vi "genMotionSensorPacket.vi"(10 "node ID":u8, 11 "state":bool) -> (3 "packet string":string)   [LabVIEW 2011]
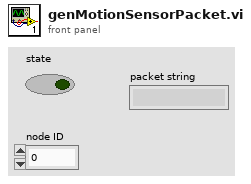
[diagram p1: front panel]
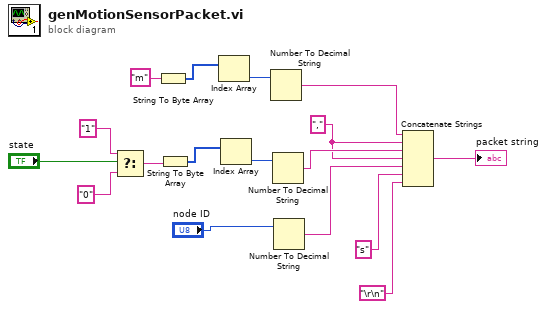
[diagram p0: block diagram]
diagram:
  w5 = ","
  n1 = Select(t="1", s="state", f="0") -> (s? t:f=w9:string)
  n2 = String To Byte Array(string="m") -> (unsigned byte array=w16:u8[])
  n3 = String To Byte Array(string=w9) -> (unsigned byte array=w13:u8[])
  n4 = Index Array(array=w16) -> (element=w15:u8)  [unwired: 1 in]
  n5 = Index Array(array=w13) -> (element=w14:u8)  [unwired: 1 in]
  n6 = Number To Decimal String(number=w15) -> (decimal integer string=w7:string)  [unwired: 1 in]
  n7 = Number To Decimal String(number=w14) -> (decimal integer string=w6:string)  [unwired: 1 in]
  n8 = Number To Decimal String(number="node ID") -> (decimal integer string=w4:string)  [unwired: 1 in]
  n9 = Concatenate Strings(w7, w5, w6, w5, w4, "s", "\r\n") -> (→"packet string":string)
